vi "CSM - Timestamp to API String Arguments.vi"(7 "Format (Empty to Use UTC)":string, 8 "Error in":errorcluster caption="Error in (no error)", 11 "Timestamp (now)":timestamp) -> (0 "Error out":errorcluster, 3 "API String":string)   [LabVIEW 2017, in "API String Arguments Support.lvlib"]
doc: "Converts a LabVIEW timestamp to an API String.\n\n-- <b>Controls</b> --\n- <b>Timestamp (now)</b>: Input timestamp. The default is the current time.\n- <b>Format(Empty to use UTC)</b>: Time format string. Uses UTC format if empty.\n\n-- <b>Indicators</b> --\n- <b>API String</b>: Converted API String format."
uses:
  API String Arguments Support.lvlib
  <userlib>/_NEVSTOP/Communicable State Machine(CSM)/_Shared/CSM Shared.lvlib
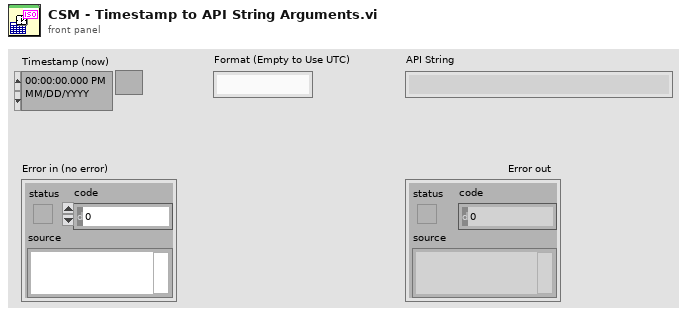
[diagram p1: front panel]
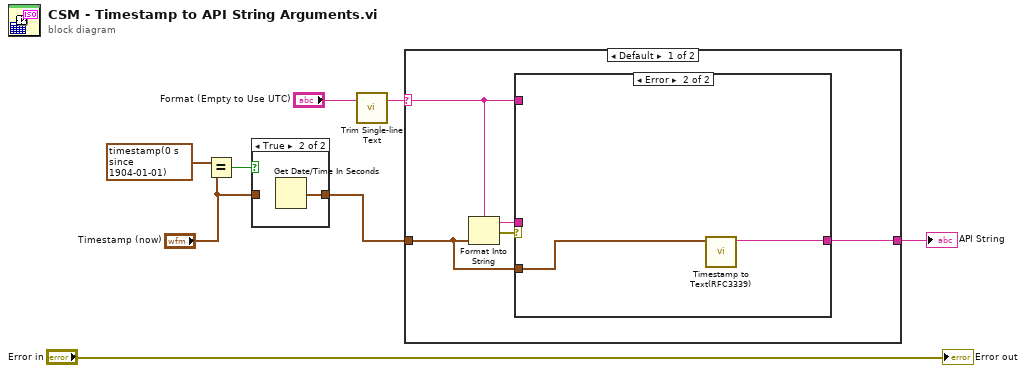
[diagram p0: block diagram]
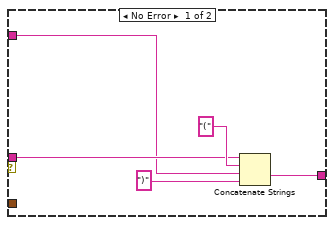
[diagram p3: hidden frame]
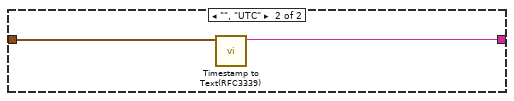
[diagram p4: hidden frame]
diagram:
  n1 = Equal?(x=timestamp(0 s since 1904-01-01), y="Timestamp (now)") -> (x = y?=w4:bool)
  n2 = case shown="True" w4 {
    tunnel: [w9 w10] -> w2
    tunnel: "Timestamp (now)" -> [w9 _]
    frame False {
    }
    frame True {
      n3 = Get Date/Time In Seconds() -> (seconds since 1Jan1904=w10:timestamp)
    }
  }
  n4 = call <userlib>:"Trim Single-line Text.vi"("single-line text"="Format (Empty to Use UTC)") -> ("trimed text"=w6:string)  [unwired: 2 in]
  n5 = case shown="Default" w6 {
    selector: w6 -> [w14 _]
    tunnel: w2 -> [w11 w24]
    tunnel: [w13 w23] -> w8
    frame Default {
      n6 = Format Into String(format string=w14, w11) -> (resulting string=w15:string, error out=w12:errorcluster)  [unwired: 2 in]
      n7 = case shown="Error" w12 {
        tunnel: w15 -> [w18 _]
        tunnel: w14 -> [w17 _]
        tunnel: [w16 w21] -> w13
        tunnel: w11 -> [_ w22]
        frame No Error {
          n8 = Concatenate Strings(w18, "(" ("string"), w17, ")" ("string")) -> (w16:string)
        }
        frame Error {
          n9 = call "Timestamp to Text(RFC3339).vi"("Time Stamp"=w22) -> ("Timestamp (RFC3339)"=w21:string)  [unwired: 9 in, 1 out]
        }
      }
    }
    frame "", "UTC" {
      n10 = call "Timestamp to Text(RFC3339).vi"("Time Stamp"=w24) -> ("Timestamp (RFC3339)"=w23:string)  [unwired: 9 in, 1 out]
    }
  }
  "API String" <- w8
  "Error out" <- "Error in"
